vi "sensor cmd sync set.vi"(10 "new_value":cluster{}, 11 "device_handle":u32) -> (2 "function return":i32, 3 "device_handle out":u32)   [LabVIEW 2019, in "apdm.lvlib"]
doc: "APDM_EXPORT int apdm_sensor_cmd_sync_set(apdm_device_handle_t device_handle, const uint64_t new_value);"
uses:
  apdm.lvlib
  Lee Lab/CP FES Walking 2018/Code/Working/LabVIEW/apdm.dll
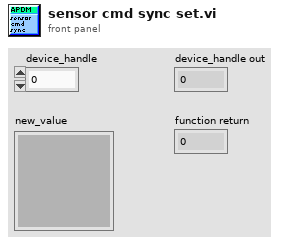
[diagram p1: front panel]
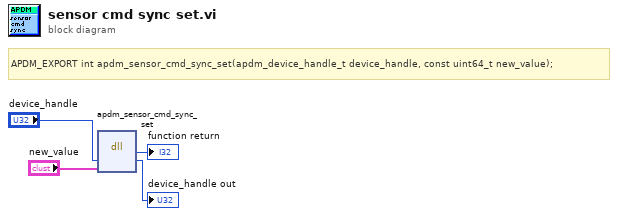
[diagram p0: block diagram]
diagram:
  # "APDM_EXPORT int apdm_sensor_cmd_sync_set(apdm_device_handle_t device_handle, const uint64_t new_value);"
  n1 = dll-call lib="C:/Users/jfalesi/Dropbox/Lee Lab/CP FES Walking 2018/Code/Working/LabVIEW/apdm.*" fn="apdm_sensor_cmd_sync_set"("device_handle"="device_handle", "new_value"="new_value") -> (→"function return":i32, "device_handle"=→"device_handle out":u32)  [unwired: 4 in, 2 out]
